vi "IsSessionLoaded.vi"(8 "error in (no error)":errorcluster, 11 "session id in":i32) -> (0 "error out":errorcluster, 2 "Is Loaded":bool, 3 "session id out":i32)   [LabVIEW 2017, in "libonnx_wrapper.lvlib"]
doc: "/**\n * @brief Проверить, загружена ли сессия в память\n * \n * Функция возвращает текущий статус сессии. Полезно для проверки перед вызовом\n * инференса, особенно если использовалась функция UnloadSession.\n * \n * @param sessionId [IN] ID сессии, полученный от CreateSession\n * \n * @return int32: 1 если сессия активна и модель загружена в память\n * @return int32: 0 если сессия не найдена или выгружена из памяти\n */\nint IsSessionLoaded(int sessionId);"
uses:
  libonnx_wrapper.lvlib
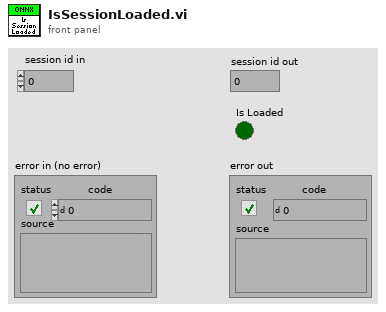
[diagram p1: front panel]
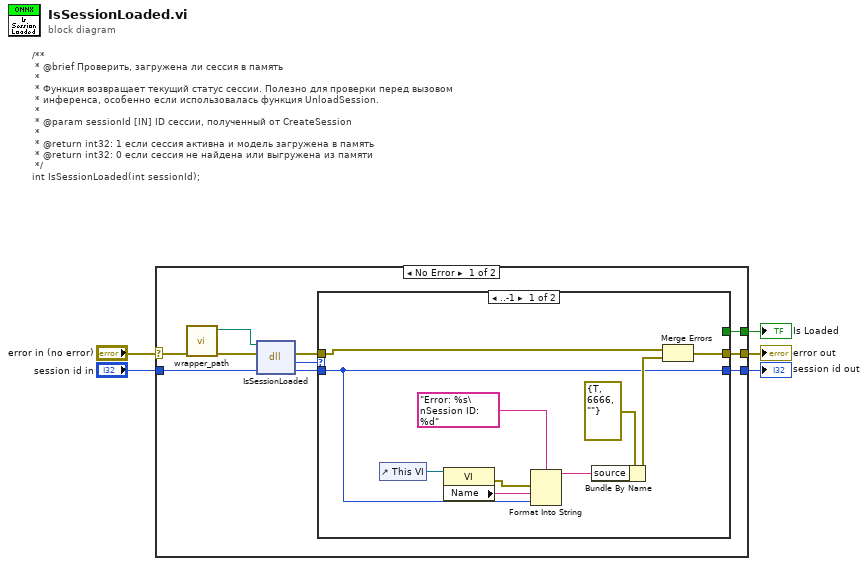
[diagram p0: block diagram]
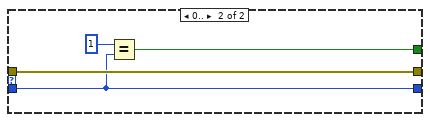
[diagram p2: hidden frame]
diagram:
  # "/**\n * @brief Проверить, загружена ли сессия в память\n * \n * Функция возвращает текущий статус сессии. Полезно для проверки перед вызовом\n * инференса, особенно если использовалась функция UnloadSession.\n * \n * @param sessionId [IN] ID сессии, полученный от CreateSession\n * \n * @return int32: 1 если сессия активна и модель загружена в память\n * @return int32: 0 если сессия не найдена или выгружена из памяти\n */\nint IsSessionLoaded(int sessionId);"
  n1 = case shown="No Error" "error in (no error)" {
    selector: "error in (no error)" -> [w6 w31]
    tunnel: "session id in" -> [w13 w30]
    tunnel: [w9 w31] -> w4
    tunnel: [w8 w30] -> w3
    tunnel: [w7 _] -> w2
    frame No Error {
      n2 = call "wrapper_path.vi"("error in (no error)"=w6) -> ("error out"=w15:errorcluster, "wrapper path"=w14:path)  [unwired: 9 in]
      n3 = dll-call lib="home/ivan/LabVIEWData/ONNX/Test/libonnx_wrapper/unix64/libonnx_wrapper.so" fn="IsSessionLoaded"(path in=w14, error in=w15, "sessionId"=w13) -> (error out=w12:errorcluster, "return"=w11:i32, "sessionId"=w10:i32)  [unwired: 1 in, 1 out]
      n4 = case shown="..-1" w11 {
        tunnel: w12 -> [w16 w29]
        tunnel: [w17 w29] -> w9
        tunnel: w10 -> [w18 w28]
        tunnel: [w18 w28] -> w8
        tunnel: [_ w26] -> w7
        frame ..-1 {
          n5 = control-ref of="This VI"() -> (w22:refnum<vi>)
          n6 = property class="VI"(reference=w22) -> (error out=w19:errorcluster, "Name"=w21:string)  [unwired: 1 in, 1 out]
          n7 = Format Into String(format string="Error: %s\nSession ID: %d", error in=w19, w21, w18) -> (resulting string=w23:string)  [unwired: 1 in, 1 out]
          n8 = Bundle By Name(cluster=errorcluster {"status"=TRUE, "code"=6666, "source"=""} ("error out"), "source"=w23) -> (w24:errorcluster)
          n9 = Merge Errors(w16, w24) -> (w17:errorcluster)
        }
        frame 0.. {
          n10 = Equal?(x=1, y=w28) -> (x = y?=w26:bool)
        }
      }
    }
    frame Error {
    }
  }
  "error out" <- w4
  "session id out" <- w3
  "Is Loaded" <- w2
